vi "Format Markdown Paragraph.vi"(8 "Error In":errorcluster, 11 "Unformatted Paragraph Input":string) -> (0 "Error Out":errorcluster, 3 "Formatted Sentence Output":string)   [LabVIEW 2017]
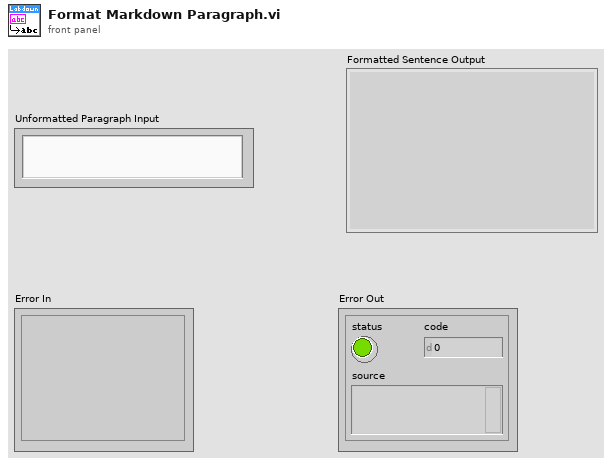
[diagram p1: front panel]
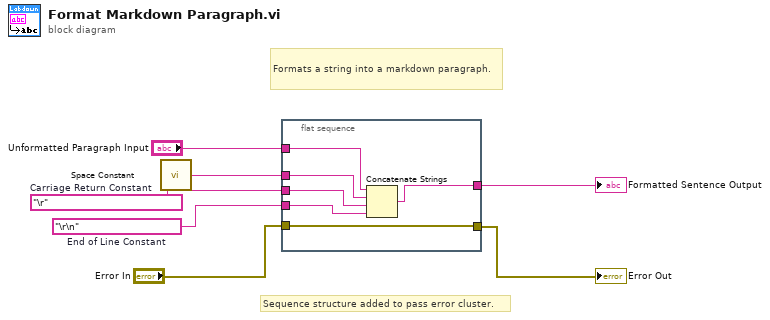
[diagram p0: block diagram]
diagram:
  w1 = "\r\n"  # End of Line Constant
  w2 = "\r"  # Carriage Return Constant
  # "Sequence structure added to pass error cluster."
  # "Formats a string into a markdown paragraph."
  n1 = call <vilib>:"Space Constant.vi"() -> ("String"=w6:string)
  n2 = flat-sequence {
    tunnel: "Unformatted Paragraph Input" -> [w13]
    tunnel: w6 -> [w12]
    tunnel: w1 -> [w8]
    tunnel: [w11] -> w5
    tunnel: "Error In" -> [w10]
    tunnel: [w10] -> w3
    tunnel: w2 -> [w9]
    frame #0 {
      n3 = Concatenate Strings(w13, w12, w9, w8) -> (w11:string)
    }
  }
  "Formatted Sentence Output" <- w5
  "Error Out" <- w3
